vi "voorbeeld sliders status.vi"() -> ()   [LabVIEW 2014]
panel:
  out "Status":string
  in  "stop":bool
  in  "Slide":dbl(slide) scale=-5.0..5.0
  out "Tank":cluster{dbl, dbl}(slide) scale=-5.0..5.0 scale format="%#.2g"
  # "Make in the properties appearance \n    Slider 1 with \"Fill from value below\"\n    Slider 2 with \"no fill\""
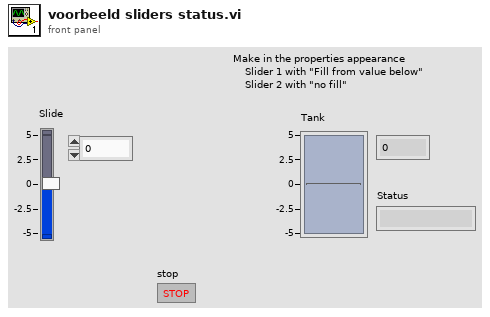
[diagram p1: front panel]
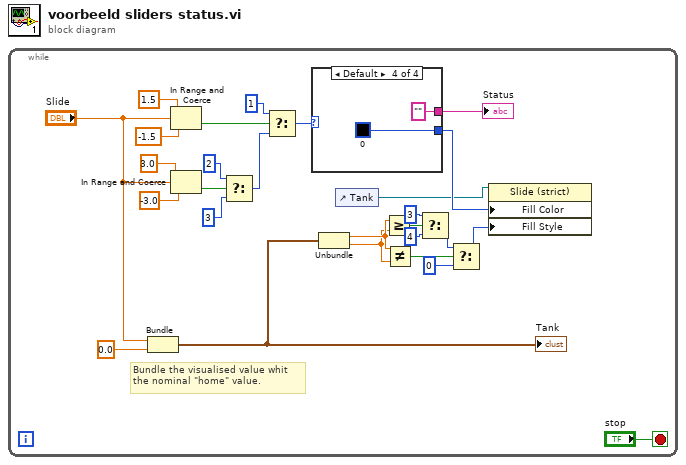
[diagram p0: block diagram]
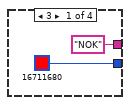
[diagram p2: hidden frame]
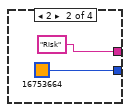
[diagram p3: hidden frame]
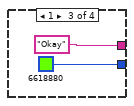
[diagram p4: hidden frame]
diagram:
  n1 = while {
    stop <- "stop" stop-if-true
    # "Bundle the visualised value whit \nthe nominal \"home\" value."
    n2 = Bundle("Slide"="Slide", 0.0) -> (w6:cluster{"Slide":dbl, dbl})  [unwired: 1 in]
    "Tank" <- w6
    n3 = In Range and Coerce(upper limit=1.5, x="Slide", lower limit=-1.5) -> (In Range?=w16:bool)  [unwired: 1 out]
    n4 = In Range and Coerce(upper limit=3.0, x="Slide", lower limit=-3.0) -> (In Range?=w14:bool)  [unwired: 1 out]
    n5 = Select(t=i16 2, s=w14, f=i16 3 ("t")) -> (s? t:f=w12:i16)
    n6 = Select(t=i16 1, s=w16, f=w12) -> (s? t:f=w10:i16)
    n7 = case shown="Default" w10 {
      tunnel: [u32 16711680 u32 16753664 u32 6618880 u32 0] -> w9
      tunnel: ["NOK" ("Status") "Risk" ("Status") "Okay" ("Status") "" ("Status")] -> w1
      frame 3 {
      }
      frame 2 {
      }
      frame 1 {
      }
      frame Default {
      }
    }
    "Status" <- w1
    n8 = Unbundle(w6) -> ("Slide"=w5:dbl, w4:dbl)
    n9 = control-ref of="Tank"() -> (w8:refnum<vi>)
    n10 = Greater Or Equal?(x=w5, y=w4) -> (x >= y?=w21:bool)
    n11 = Not Equal?(x=w5, y=w4) -> (x != y?=w25:bool)
    n12 = Select(t=3, s=w21, f=4) -> (s? t:f=w24:i32)
    n13 = Select(t=w24, s=w25, f=0) -> (s? t:f=w27:i32)
    n14 = property on="Property Node" class="Slide (strict)"(reference=w8, "Fill Color"=w9, "Fill Style"=w27) -> ()  [unwired: 1 in, 2 out]
  }
